vi "Gen - Decimal Place.vi"(11 "DigNum Refnum":refnum<vi>) -> ()   [LabVIEW 2019]
uses:
  Controls/FGV States.ctl
panel:
  out "error out":errorcluster
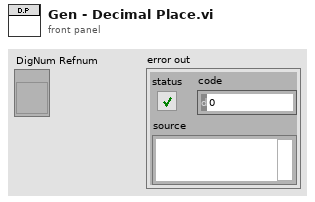
[diagram p1: front panel]
types:
  T1 = typedef "FGV States.ctl" = enum16{"Read", "Write"}
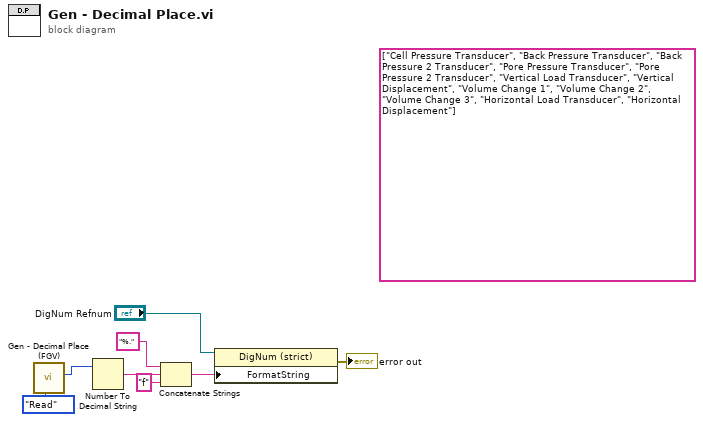
[diagram p0: block diagram]
diagram:
  (unwired) string[] ["Cell Pressure Transducer", "Back Pressure Transducer", "Back Pressure 2 Transducer", "Pore Pressure Transducer", "Pore Pressure 2 Transducer", "Vertical Load Transducer", "Vertical Displacement", "Volume Change 1", "Volume Change 2", "Volume Change 3", "Horizontal Load Transducer", "Horizontal Displacement"] ("Array")
  n1 = call "Gen - Decimal Place (FGV).vi"("Action"=FGV_States."Read") -> ("Ch2 out"=w1:u8)  [unwired: 8 in, 2 out]
  n2 = Number To Decimal String(number=w1) -> (decimal integer string=w8:string)  [unwired: 1 in]
  n3 = Concatenate Strings("%." ("Format String"), w8, "f" ("string")) -> (w5:string)
  n4 = property on="Property Node" class="DigNum (strict)"(reference="DigNum Refnum", "FormatString"=w5) -> (error out=→"error out":errorcluster)  [unwired: 1 in, 1 out]
